vi "AO Referenece.vi"(8 "error in (no error)":errorcluster, 11 "Item Ref in":T1 format="%.0x") -> (0 "error out":errorcluster, 1 "AO Refs":T1[](array[typedef]) format="%.0x", 2 "AO Refs":T2(array[cluster]) {"VS Refs" format="%.0x"}, 3 "Item Ref out":T1 format="%.0x")   [LabVIEW 2021, in "DAQ Analog InOut System Explorer.lvlib"]
uses:
  DAQ Analog InOut System Explorer.lvlib
  <vilib>/NI VeriStand/Custom Device API/Custom Device API.lvlib
  <vilib>/NI VeriStand/Custom Device API/Custom Device Item Ref.ctl
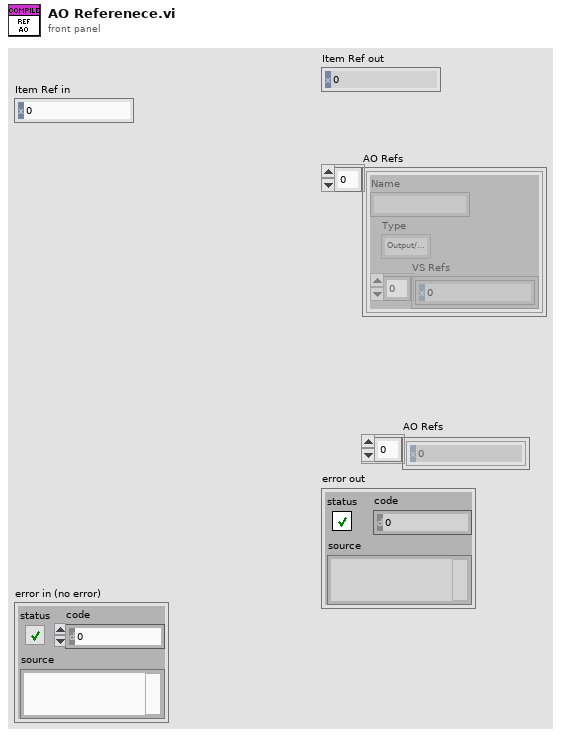
[diagram p1: front panel]
types:
  T1 = typedef "Custom Device API.lvlib/Custom Device Item Ref.ctl" = u64
  T2 = cluster{"Name":string, "Type":enum16{"Output/Write", "Input/Read", "Input/ReadWrite"}, "VS Refs":T1[]}[]
  T3 = enum16{"Output/Write", "Input/Read", "Input/ReadWrite"}
  T4 = cluster{"Name":string, "Type":enum16{"Output/Write", "Input/Read", "Input/ReadWrite"}, "VS Refs":T1[]}
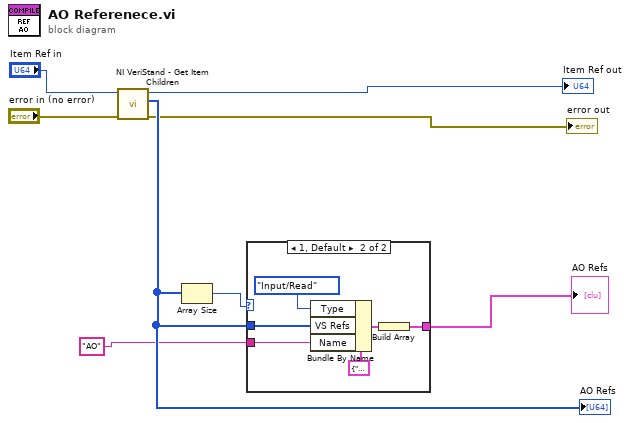
[diagram p0: block diagram]
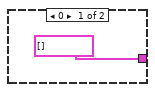
[diagram p2: hidden frame]
diagram:
  n1 = call <vilib>:"NI VeriStand - Get Item Children.vi"("error in (no error)"="error in (no error)", "Item Ref in"="Item Ref in") -> ("error out"=→"error out":errorcluster, "Child Refs"=w8:T1[], "Item Ref out"=→"Item Ref out":T1)  [unwired: 6 in, 1 out]
  "AO Refs" <- w8
  n2 = Array Size(array=w8) -> (size(s)=w7:i32)
  n3 = case shown="1, Default" w7 {
    tunnel: w8 -> [_ w13]
    tunnel: [T2 [] w11] -> w1
    tunnel: "AO" ("Name") -> [_ w10]
    frame 0 {
    }
    frame 1, Default {
      n4 = Bundle By Name(cluster=T4 {"Name"="", "Type"=enum."Output/Write", "VS Refs"=[]} ("Group"), "Type"=T3."Input/Read", "VS Refs"=w13, "Name"=w10) -> (w12:T4)
      n5 = Build Array(w12) -> (w11:T2)
    }
  }
  "AO Refs" <- w1
